vi "例程47-移位寄存器的使用.vi"() -> ()   [LabVIEW 2016]
panel:
  out "波形图表 2":dbl[](graph)
  in  "停止":bool
  out "波形图表":dbl(graph)
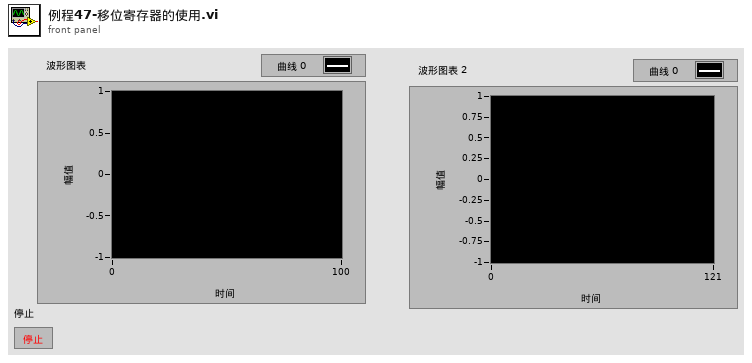
[diagram p1: front panel]
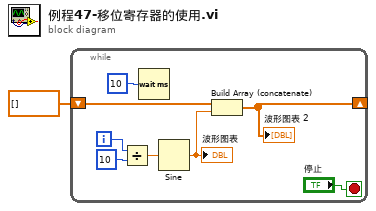
[diagram p0: block diagram]
diagram:
  n1 = while {
    shift-right: [w5] -> _
    shift-left: dbl[] [] -> [w8]
    i -> [w3]
    stop <- "停止" stop-if-true
    n2 = Divide(x=w3, y=10) -> (x/y=w4:dbl)
    n3 = Wait (ms)(milliseconds to wait=u32 10 ("等待时间（毫秒）")) -> ()  [unwired: 1 out]
    n4 = Sine(x=w4) -> (sin(x)=w7:dbl)
    "波形图表" <- w7
    n5 = Build Array (concatenate)(w8, w7) -> (w5:dbl[])
    "波形图表 2" <- w5
  }
